vi "Array_Image.vi"() -> ()   [LabVIEW 2022 SP3]
uses:
  <vilib>/addons/_jki/python_bridge/Server/Server.lvclass
panel:
  out "JSON string 2":string
  out "error out 2":errorcluster
  out "Python Connected":bool
  in  "Send to Python":bool
  out "size(s)":i32[](array[numeric])
  out "Array":dbl[][](array[numeric])
  in  "Connect to Python":bool
  in  "Clear":bool
  in  "Stop":bool
  out "Draw pane":picture
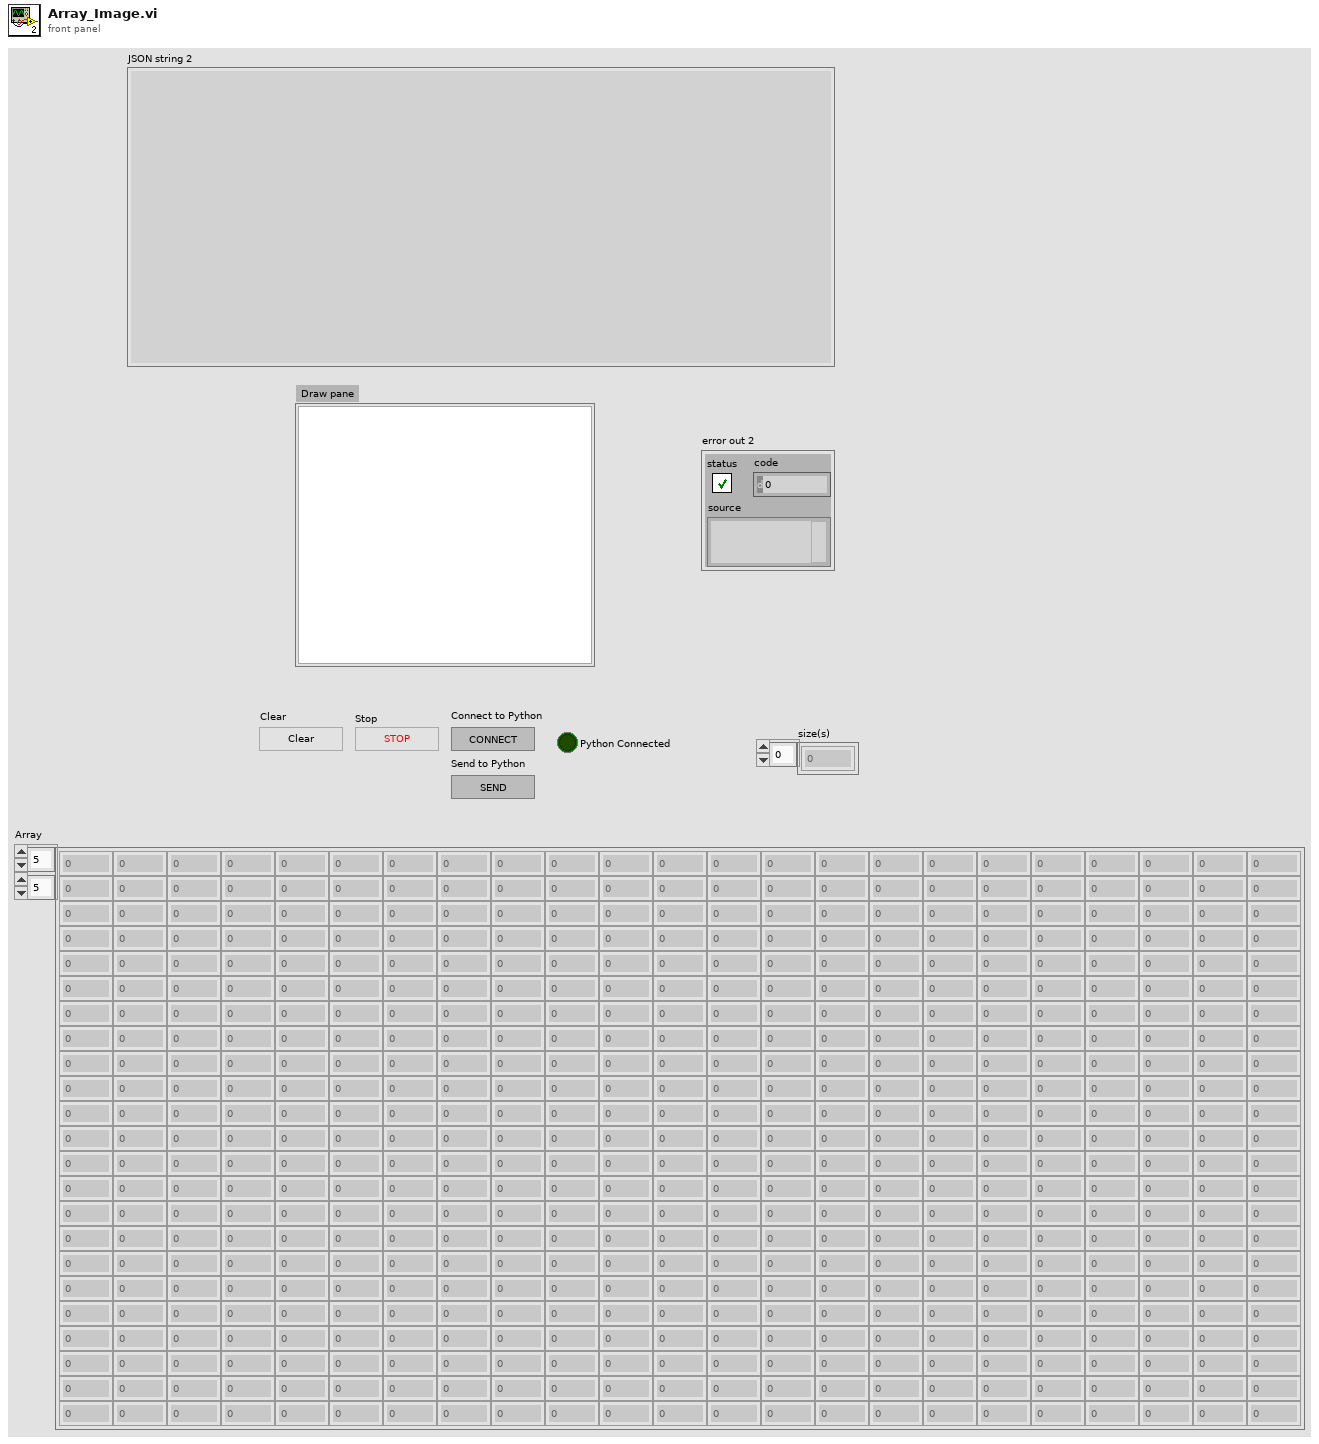
[diagram p1: front panel]
types:
  T1 = cluster{"Width":u16, "Style":enum32{"Solid", "Dash", "Dot", "DashDot", "DashDotDot"}}
  T2 = typedef "LVMouseTypeDef.ctl" = cluster{"Mouse Position":cluster{"X":i32, "Y":i32}, "Mouse Modifiers":cluster{"Button Down":bool, "Shift Mod":bool, "Menu Mod":bool, "Option Mod":bool}}
  T3 = cluster{"Button Down":bool, "Shift Mod":bool, "Menu Mod":bool, "Option Mod":bool}
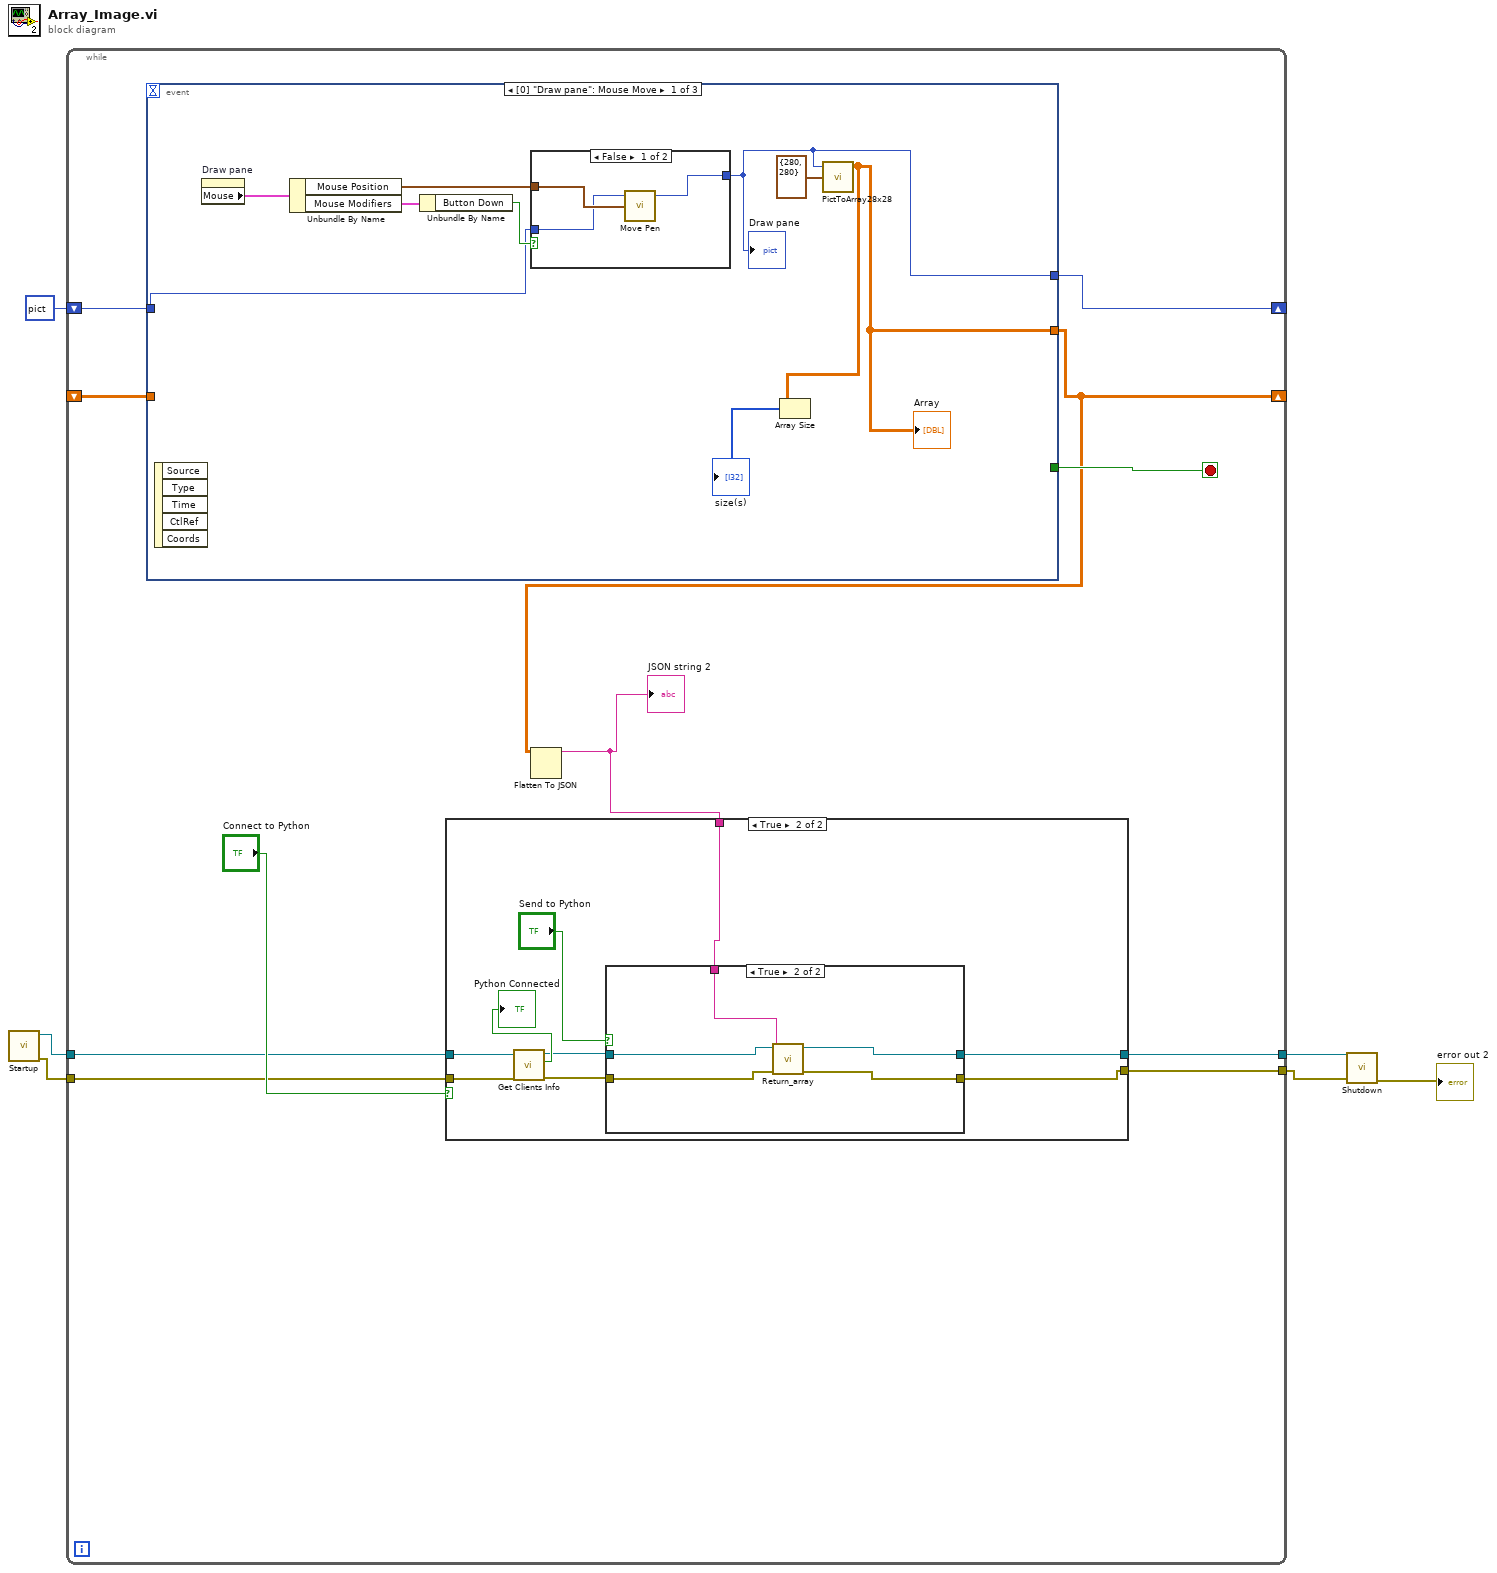
[diagram p0: block diagram]
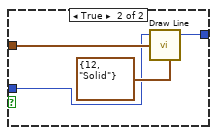
[diagram p4: hidden frame]
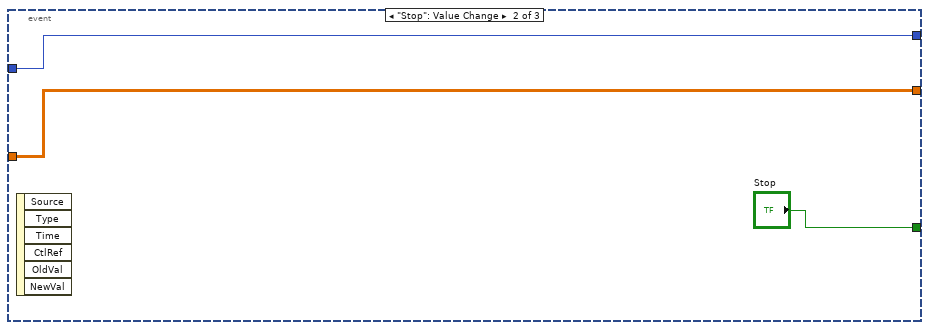
[diagram p5: hidden frame]
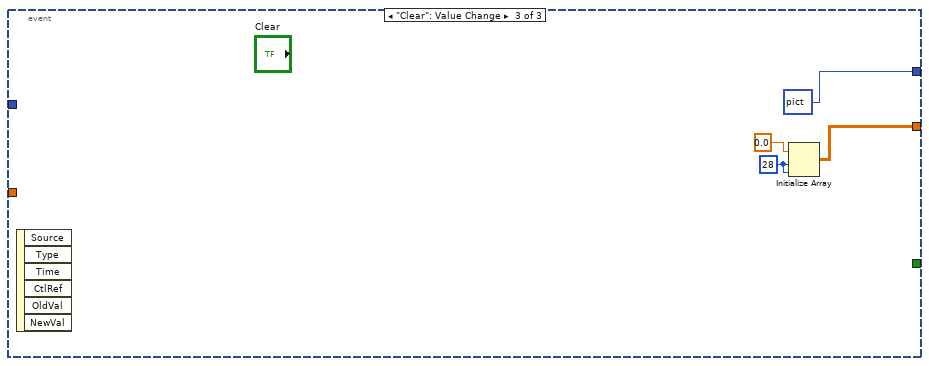
[diagram p6: hidden frame]
diagram:
  n1 = call <vilib>:"Startup.vi"() -> ("error out"=w2:errorcluster, "JKI_Python_Server out"=w1:refnum<class "Server.lvclass">)  [unwired: 10 in]
  n2 = while {
    shift-right: [w17] -> _
    shift-left: picture data[5B] ("empty picture") -> [w16]
    shift-right: [w12] -> _
    shift-left: _ -> [w14]
    tunnel: [w10] -> w5
    tunnel: [w9] -> w4
    tunnel: w2 -> [w8]
    tunnel: w1 -> [w7]
    stop <- w15 stop-if-true
    n3 = event shown="[0] \"Draw pane\": Mouse Move" {
      selector: _ -> [_ _ _]
      dyn-events: _ -> [_ _ _]
      timeout: _ -> [_ _ _]
      tunnel: [w38 w53 picture data[5B] ("empty picture")] -> w17
      tunnel: w16 -> [w40 w53 _]
      tunnel: [_ "Stop" _] -> w15
      tunnel: [w36 w52 w55] -> w12
      tunnel: w14 -> [_ w52 _]
      event "Draw pane": Mouse Move {
        n4 = event-data() -> ()  [unwired: 1 in, 5 out]
        n5 = property on="Draw pane" class="Pict"() -> ("Mouse"=w44:T2)  [unwired: 2 in, 2 out]
        n6 = Unbundle By Name(w44) -> ("Mouse Position"=w42:cluster{"X":i32, "Y":i32}, "Mouse Modifiers"=w43:T3)
        n7 = Unbundle By Name(w43) -> ("Button Down"=w41:bool)
        n8 = case shown="False" w41 {
          tunnel: w42 -> [w46 w51]
          tunnel: [w47 w50] -> w38
          tunnel: w40 -> [w45 w48]
          frame False {
            n9 = call <vilib>:"Move Pen.vi"("new position"=w46, "picture"=w45) -> ("new picture"=w47:picture)  [unwired: 3 in]
          }
          frame True {
            n10 = call <vilib>:"Draw Line.vi"("picture"=w48, "end point"=w51, "pen"=T1 {"Width"=12, "Style"=enum."Solid"}) -> ("new picture"=w50:picture)  [unwired: 6 in]
          }
        }
        "Draw pane" <- w38
        n11 = call "PictToArray28x28.vi"("Draw Area Size"=cluster{"Width":u32, "Height":u32} {"Width"=280, "Height"=280}, "Picture"=w38) -> ("Array"=w36:dbl[][])  [unwired: 1 in, 2 out]
        "Array" <- w36
        n12 = Array Size(array=w36) -> (size(s)=→"size(s)":i32[])
      }
      event "Stop": Value Change {
        n13 = event-data() -> ()  [unwired: 1 in, 6 out]
      }
      event "Clear": Value Change {
        w56 = 28 ("dimension size")
        n14 = event-data() -> ()  [unwired: 1 in, 6 out]
        n15 = Initialize Array(sgl 0.0 ("element"), w56, w56) -> (w55:sgl[][])
      }
    }
    n16 = Flatten To JSON(anything=w12) -> (JSON string=w11:string)  [unwired: 2 in, 1 out]
    "JSON string 2" <- w11
    n17 = case shown="True" "Connect to Python" {
      tunnel: w11 -> [_ w27]
      tunnel: [w18 w26] -> w10
      tunnel: [w19 w25] -> w9
      tunnel: w8 -> [w18 w22]
      tunnel: w7 -> [w19 w23]
      frame False {
      }
      frame True {
        n18 = call <vilib>:"Get Clients Info.vi"("error in (no error)"=w22, "JKI_Python_Server in"=w23) -> ("error out"=w21:errorcluster, "Client Connected"=→"Python Connected":bool, "JKI_Python_Server out"=w20:refnum<class "Server.lvclass">)  [unwired: 5 in, 2 out]
        n19 = case shown="True" "Send to Python" {
          tunnel: w21 -> [w29 w34]
          tunnel: w20 -> [w30 w35]
          tunnel: [w30 w32] -> w25
          tunnel: [w29 w33] -> w26
          tunnel: w27 -> [_ w31]
          frame False {
          }
          frame True {
            n20 = call "Return_array.vi"("error in (no error)"=w34, "String"=w31, "JKI_Python_Server in"=w35) -> ("error IO"=w33:errorcluster, "JKI_Python_Server out"=w32:refnum<class "Server.lvclass">)  [unwired: 7 in]
          }
        }
      }
    }
  }
  n21 = call <vilib>:"Shutdown.vi"("error in (no error)"=w5, "JKI_Python_Server in"=w4) -> ("error out"=→"error out 2":errorcluster)  [unwired: 9 in]
